vi "test Scheduled Loopback with Disable.vi"(8 "error in":errorcluster, 11 "TestCase in":refnum<class "Single Board Loopback.lvclass">) -> (0 "error out":errorcluster, 3 "TestCase out":refnum<class "Single Board Loopback.lvclass">)   [LabVIEW 2020, in "Single Board Loopback.lvclass"]
uses:
  Single Board Loopback.lvclass
  C:/dev/git/niveristand-custom-device-testing-tools/VeriStandTestCase/VeriStandTestCase.lvclass
  <vilib>/numeric/Random Number (Range) U64.vi
  <vilib>/numeric/sub_Random U32.vi
  <vilib>/NI VeriStand/Execution/Workspace/NI VeriStand - Set Multiple Channel Values.vi
  <vilib>/addons/_JKI Toolkits/VI Tester/TestCase.llb/TestCase.lvclass
  niveristand-custom-device-testing-tools/VeriStandTestUtilities/VeriStandTestUtilities.lvlib
  <vilib>/NI VeriStand/Execution/Workspace/NI_VS Workspace ExecutionAPI.lvlib
  C:/Program Files (x86)/National Instruments/LabVIEW 2020/vi.lib/addons/_JKI Toolkits/VI Tester/TestCase.llb/TestCase.lvclass
  C:/dev/git/niveristand-aim-arinc429-custom-device/Source/Custom Device Support/Tests/System/Single Board Loopback/Single Board Loopback.lvclass
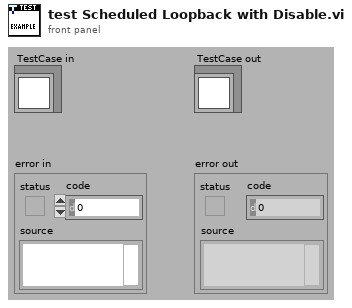
[diagram p1: front panel]
types:
  T1 = typedef "NI_VS Workspace ExecutionAPI.lvlib/WorkspaceAPI.ctl" = refnum<k24>
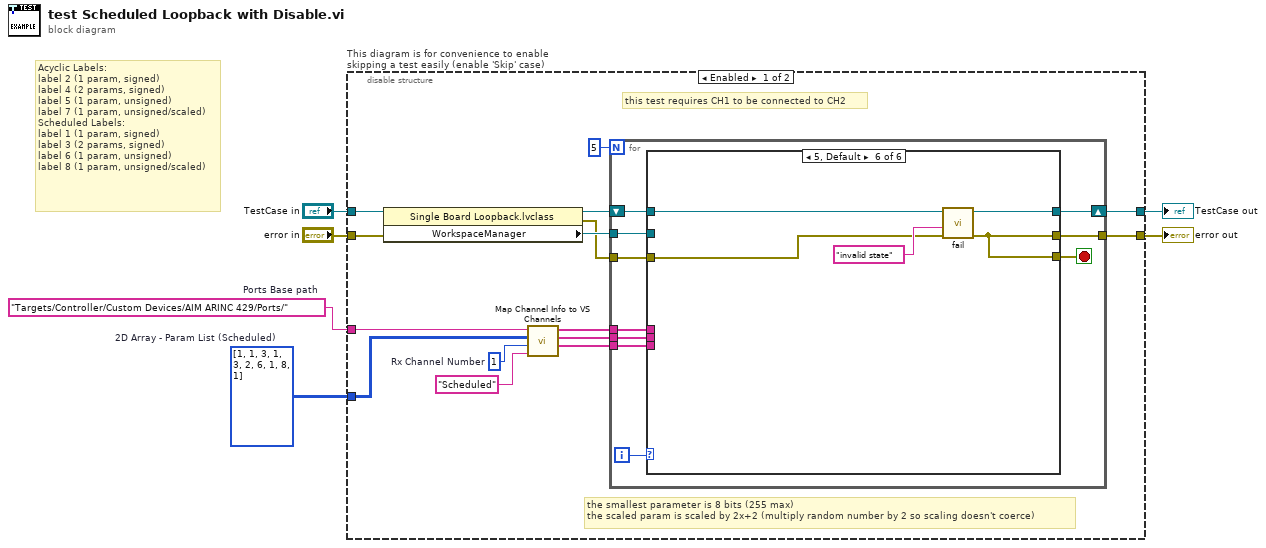
[diagram p0: block diagram]
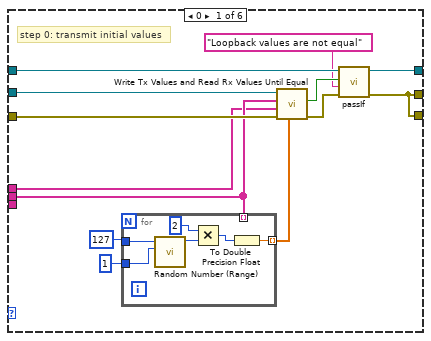
[diagram p2: hidden frame]
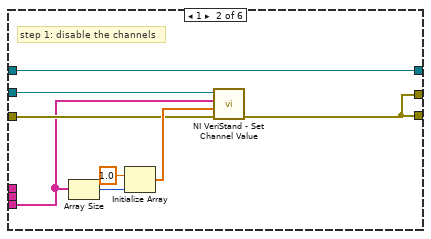
[diagram p3: hidden frame]
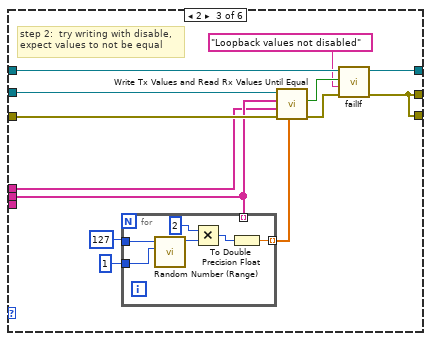
[diagram p4: hidden frame]
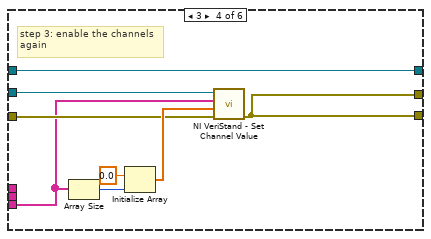
[diagram p5: hidden frame]
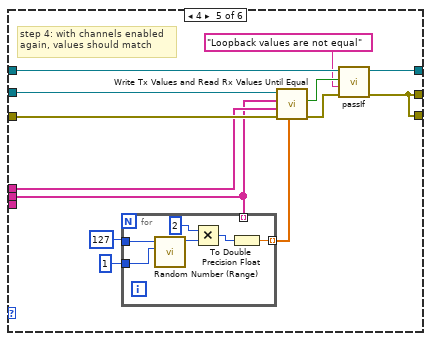
[diagram p6: hidden frame]
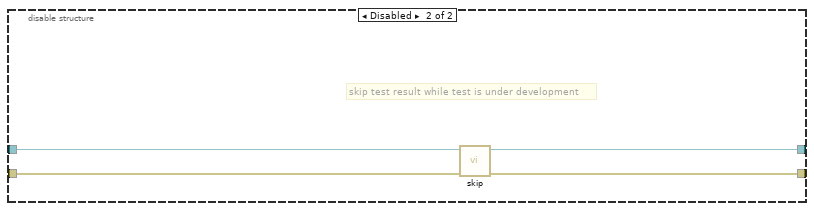
[diagram p7: hidden frame]
diagram:
  w1 = i32[][] [[1, 1], [3, 1], [3, 2], [6, 1], [8, 1]]  # 2D Array - Param List (Scheduled)
  w2 = "Targets/Controller/Custom Devices/AIM ARINC 429/Ports/"  # Ports Base path
  # "Acyclic Labels:\nlabel 2 (1 param, signed)\nlabel 4 (2 params, signed)\nlabel 5 (1 param, unsigned)\nlabel 7 (1 param, unsigned/scaled)\nScheduled Labels:\nlabel 1 (1 param, signed)\nlabel 3 (2 params, signed)\nlabel 6 (1 param, unsigned)\nlabel 8 (1 param, unsigned/scaled)"
  n1 = disable-structure "This diagram is for convenience to enable skipping a test easily (enable 'Skip' case)" shown="Enabled" {
    disable-tunnel: "TestCase in" -> [w16 w113]
    disable-tunnel: [w14 w111] -> w3
    disable-tunnel: [w13 w112] -> w5
    disable-tunnel: "error in" -> [w15 w110]
    disable-tunnel: w2 -> [w17 _]
    disable-tunnel: w1 -> [w10 _]
    frame Enabled {
      w11 = 1  # Rx Channel Number
      # "this test requires CH1 to be connected to CH2"
      # "the smallest parameter is 8 bits (255 max)\nthe scaled param is scaled by 2x+2 (multiply random number by 2 so scaling doesn't coerce)"
      n2 = property class="Single Board Loopback.lvclass"(reference=w16, error in=w15) -> (reference out=w18:refnum<class "Single Board Loopback.lvclass">, error out=w19:errorcluster, "WorkspaceManager"=w20:T1)
      n3 = call "Map Channel Info to VS Channels.vi"("Transfer Type"="Scheduled", "Rx Channel Number"=w11, "2D Array - Label/Param List"=w10, "VS Channel Base Port"=w17) -> ("Tx Disable Channels Array"=w8:string[], "Tx Channels Array"=w9:string[], "Rx Channels Array"=w21:string[])  [unwired: 4 in, 1 out]
      n4 = for {
        N: 5 -> [_]
        tunnel: w21 -> [w31]
        tunnel: w20 -> [w30]
        tunnel: w19 -> [w29]
        tunnel: w9 -> [w25]
        shift-right: [w27] -> w14
        shift-left: w18 -> [w28]
        tunnel: [w26] -> w13
        tunnel: w8 -> [w22]
        i -> [w24]
        stop <- w23 stop-if-true
        n5 = case shown="5, Default" w24 {
          tunnel: w31 -> [w32 _ w59 _ w87 _]
          tunnel: w30 -> [w44 w54 w71 w81 w98 _]
          tunnel: w29 -> [w43 w53 w70 w80 w97 w106]
          tunnel: w28 -> [w41 w58 w68 w85 w95 w108]
          tunnel: [w40 w58 w67 w85 w94 w109] -> w27
          tunnel: [w34 w52 w61 w79 w88 w105] -> w26
          tunnel: w25 -> [w33 _ w60 _ w86 _]
          tunnel: [w34 w52 w61 w79 w88 w105] -> w23
          tunnel: w22 -> [_ w51 _ w78 _ _]
          frame 0 {
            # "step 0: transmit initial values"
            n6 = for {
              tunnel: [w49] -> w35 mode=indexing
              tunnel: u64 127 ("upper bound (100)") -> [w48]
              tunnel: u64 1 ("upper bound (100)") -> [w47]
              tunnel: w33 -> [_] mode=indexing
              n7 = call-poly <vilib>:"Random Number (Range).vi"("lower bound (0)"=w47, "upper bound (100)"=w48) -> ("number"=w50:u64)  [unwired: 9 in]
              n8 = Multiply(x=u64 2, y=w50) -> (x*y=w46:u64)
              n9 = To Double Precision Float(number=w46) -> (double precision float=w49:dbl)
            }
            n10 = call "Write Tx Values and Read Rx Values Until Equal.vi"("Tx values"=w35, "error in"=w43, "Rx aliases"=w32, "Tx aliases"=w33, "workspace manager in"=w44) -> ("error out"=w42:errorcluster, "values equal"=w39:bool)  [unwired: 4 in, 1 out]
            n11 = call-dynamic "passIf.vi"("error in (no error)"=w42, "message (\"\")"="Loopback values are not equal" ("message (\"\")"), "pass"=w39, "TestCase in"=w41) -> ("error out"=w34:errorcluster, "TestCase out"=w40:refnum<class "Single Board Loopback.lvclass">)  [unwired: 6 in]
          }
          frame 1 {
            # "step 1: disable the channels"
            n12 = Array Size(array=w51) -> (size(s)=w57:i32)
            n13 = Initialize Array(1.0 ("element"), w57) -> (w55:dbl[])
            n14 = call-poly <vilib>:"NI VeriStand - Set Channel Value.vi"("error in (no error)"=w53, "Values"=w55, "Channels"=w51, "WorkspaceManager in"=w54) -> ("error out"=w52:errorcluster)  [unwired: 6 in, 1 out]
          }
          frame 2 {
            # "step 2:  try writing with disable,\nexpect values to not be equal"
            n15 = for {
              tunnel: [w76] -> w62 mode=indexing
              tunnel: u64 127 ("upper bound (100)") -> [w75]
              tunnel: u64 1 ("upper bound (100)") -> [w74]
              tunnel: w60 -> [_] mode=indexing
              n16 = call-poly <vilib>:"Random Number (Range).vi"("lower bound (0)"=w74, "upper bound (100)"=w75) -> ("number"=w77:u64)  [unwired: 9 in]
              n17 = Multiply(x=u64 2, y=w77) -> (x*y=w73:u64)
              n18 = To Double Precision Float(number=w73) -> (double precision float=w76:dbl)
            }
            n19 = call "Write Tx Values and Read Rx Values Until Equal.vi"("Tx values"=w62, "error in"=w70, "Rx aliases"=w59, "Tx aliases"=w60, "workspace manager in"=w71) -> ("error out"=w69:errorcluster, "values equal"=w66:bool)  [unwired: 4 in, 1 out]
            n20 = call-dynamic "failIf.vi"("error in (no error)"=w69, "message (\"\")"="Loopback values not disabled" ("message (\"\")"), "fail"=w66, "TestCase in"=w68) -> ("error out"=w61:errorcluster, "TestCase out"=w67:refnum<class "Single Board Loopback.lvclass">)  [unwired: 6 in]
          }
          frame 3 {
            # "step 3: enable the channels\nagain"
            n21 = Array Size(array=w78) -> (size(s)=w84:i32)
            n22 = Initialize Array(0.0 ("element"), w84) -> (w82:dbl[])
            n23 = call-poly <vilib>:"NI VeriStand - Set Channel Value.vi"("error in (no error)"=w80, "Values"=w82, "Channels"=w78, "WorkspaceManager in"=w81) -> ("error out"=w79:errorcluster)  [unwired: 6 in, 1 out]
          }
          frame 4 {
            # "step 4: with channels enabled\nagain, values should match"
            n24 = for {
              tunnel: [w103] -> w89 mode=indexing
              tunnel: u64 127 ("upper bound (100)") -> [w102]
              tunnel: u64 1 ("upper bound (100)") -> [w101]
              tunnel: w86 -> [_] mode=indexing
              n25 = call-poly <vilib>:"Random Number (Range).vi"("lower bound (0)"=w101, "upper bound (100)"=w102) -> ("number"=w104:u64)  [unwired: 9 in]
              n26 = Multiply(x=u64 2, y=w104) -> (x*y=w100:u64)
              n27 = To Double Precision Float(number=w100) -> (double precision float=w103:dbl)
            }
            n28 = call "Write Tx Values and Read Rx Values Until Equal.vi"("Tx values"=w89, "error in"=w97, "Rx aliases"=w87, "Tx aliases"=w86, "workspace manager in"=w98) -> ("error out"=w96:errorcluster, "values equal"=w93:bool)  [unwired: 4 in, 1 out]
            n29 = call-dynamic "passIf.vi"("error in (no error)"=w96, "message (\"\")"="Loopback values are not equal" ("message (\"\")"), "pass"=w93, "TestCase in"=w95) -> ("error out"=w88:errorcluster, "TestCase out"=w94:refnum<class "Single Board Loopback.lvclass">)  [unwired: 6 in]
          }
          frame 5, Default {
            n30 = call-dynamic "fail.vi"("error in (no error)"=w106, "message (\"\")"="invalid state" ("message (\"\")"), "TestCase in"=w108) -> ("error out"=w105:errorcluster, "TestCase out"=w109:refnum<class "Single Board Loopback.lvclass">)  [unwired: 7 in]
          }
        }
      }
    }
    frame Disabled {
      # "skip test result while test is under development"
      n31 = call <vilib>:"skip.vi"("error in (no error)"=w110, "TestCase in"=w113) -> ("error out"=w112:errorcluster, "TestCase out"=w111:refnum<class "Single Board Loopback.lvclass">)  [unwired: 8 in]
    }
  }
  "error out" <- w5
  "TestCase out" <- w3
